vi "LEDWrite.vi"(10 "Data To Send":u8[](array[numeric])=[66, 67, 1, 0, 0, 0, 69, 67, 0, 0], 11 "Enum":enum16{"Write", "Open"}(ring)) -> ()   [LabVIEW 2019]
uses:
  <vilib>/Rock Robotics/SystemInterfaces/spilib/spi_bus.ctl
  <vilib>/Rock Robotics/WPI/SPI/WPI_SPIMode.ctl
  Robot Global Data.vi
panel:
  out "Received Data":u8[](array[numeric])
  out "error out":errorcluster
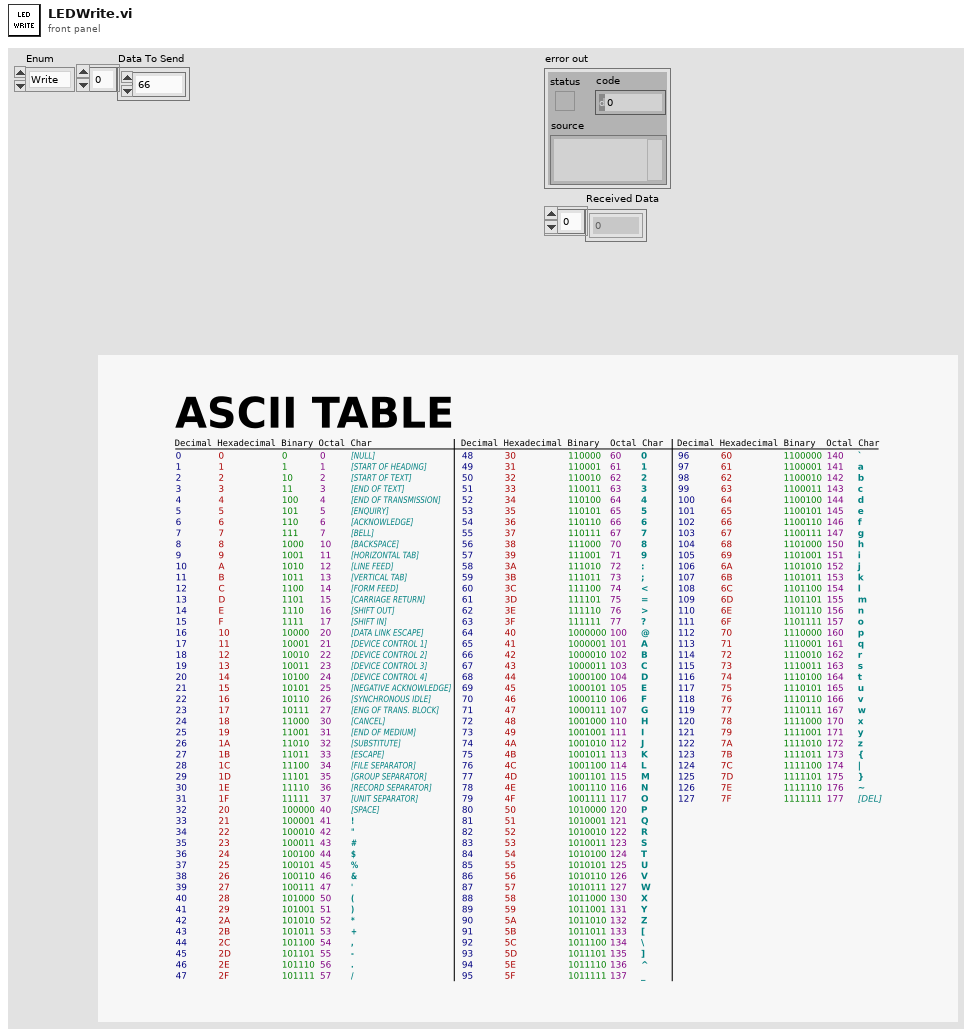
[diagram p1: front panel]
types:
  T1 = typedef "WPI_SPIMode.ctl" = enum16{"Mode 0 (Clk Idle Low,Sample on Leading)", "Mode 1 (Clk Idle Low,Sample on Trailing)", "Mode 2 (Clk Idle High,Sample on Leading)", "Mode 3 (Clk Idle High,Sample on Trailing)"}
  T2 = typedef "spi_bus.ctl" = enum16{"SPI On-Board, CS0", "SPI On-Board, CS1", "SPI On-Board, CS2", "SPI On-Board, CS3", "SPI MXP", "Invalid"}
  T3 = typedef "WPI_SPIDevRef.ctl" = cluster{"DevStatus":errorcluster, "Handle":i32, "SPI Bus":T2}
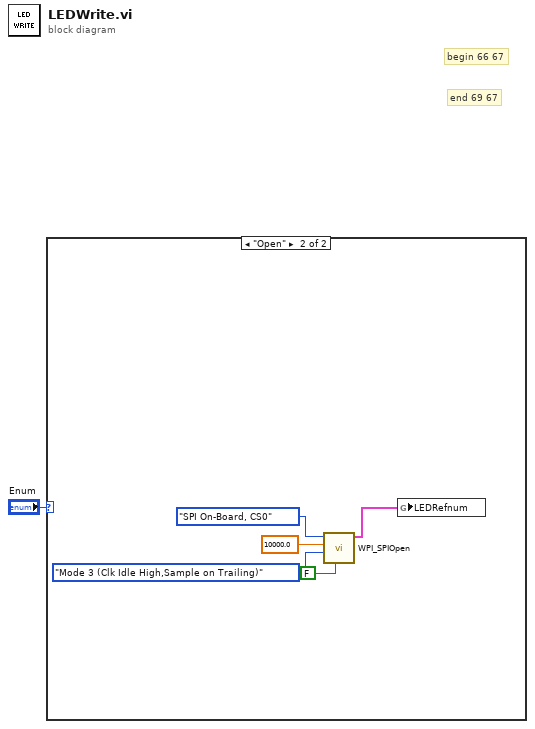
[diagram p0: block diagram]
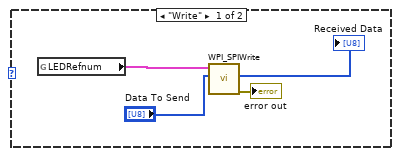
[diagram p2: hidden frame]
diagram:
  # "end 69 67"
  # "begin 66 67"
  n1 = case shown="\"Open\"" "Enum" {
    frame "Write" {
      n2 = global read "Robot Global Data.vi" "LEDRefnum"() -> (w4:T3)
      n3 = call <vilib>:"WPI_SPIWrite.vi"("Data To Send"="Data To Send", "SPIDevRef"=w4) -> ("error out"=→"error out":errorcluster, "Received Data"=→"Received Data":u8[])  [unwired: 7 in, 1 out]
    }
    frame "Open" {
      n4 = call <vilib>:"WPI_SPIOpen.vi"("Chip Select Active High (F)"=FALSE, "Mode (3)"=WPI_SPIMode."Mode 3 (Clk Idle High,Sample on Trailing)", "Clock Rate (Hz)"=10000.0, "SPI Bus"=spi_bus."SPI On-Board, CS0") -> ("SPIDevRef"=w6:T3)  [unwired: 6 in, 1 out]
      n5 = global write "Robot Global Data.vi" "LEDRefnum"(w6) -> ()
    }
  }
